vi "CompactRIO IO.vi"() -> ()   [LabVIEW 2009]
uses:
  <vilib>/eio/EIONode/EIONode.xnode
  <vilib>/rvi/eio/nirviEIOImplementation/nirviEIOImplementation.xnode
  <vilib>/rvi/eio/common/nirviEmuTemplateMethod_noerrors.vi
  <vilib>/rvi/eio/common/nirviEmuClasses.ctl
panel:
  in  "stop":bool
  out "Thermocouple Difference":fxp<+/-,25,-1> format="%.26g"
  out "Thermocouple 1":fxp<+/-,24,-2> format="%.26g"
  out "Thermocouple 0":fxp<+/-,24,-2> format="%.26g"
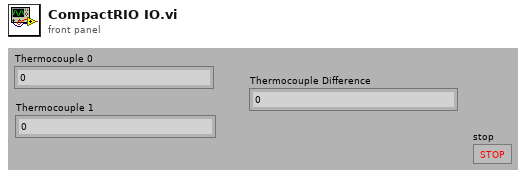
[diagram p1: front panel]
types:
  T1 = typedef "nirviEmuClasses.ctl" = enum16{"IO Read", "IO Write", "Method", "Property Read", "Property Write"}
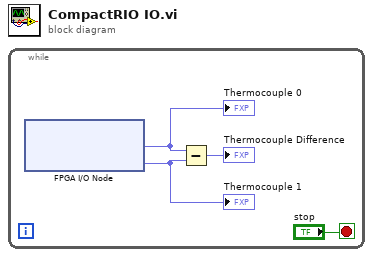
[diagram p0: block diagram]
diagram:
  n1 = while {
    stop <- "stop" stop-if-true
    n2 = xnode "FPGA I/O Node"() -> ("Thermocouple 0"=w2:fxp<+/-,24,-2>, "Thermocouple 1"=w4:fxp<+/-,24,-2>)  [unwired: 2 in, 2 out]
    "Thermocouple 0" <- w2
    "Thermocouple 1" <- w4
    n3 = Subtract(x=w2, y=w4) -> (x-y=→"Thermocouple Difference":fxp<+/-,25,-1>)
  }
